vi "Error Handler.vi"(8 "错误输入":cluster{"状态":bool, "代码":i32, "源":string}, 11 "队列输入":refnum<queue>) -> (0 "错误输出":cluster{"状态":bool, "代码":i32, "源":string}, 3 "队列输出":refnum<queue>)   [LabVIEW 2012]
doc: "该子VI监控“生产者循环”和“消费者循环”的“错误簇”连线。任意循环中出错时，该子VI向“消费者循环”发送消息以便关闭循环。"
uses:
  Consumer Message.ctl
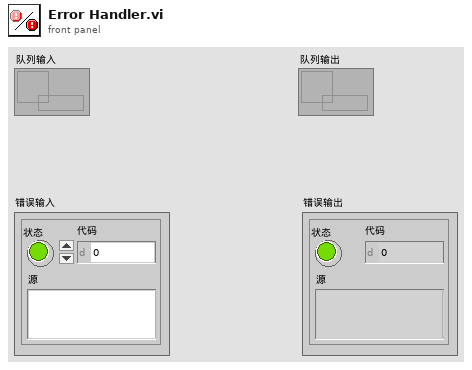
[diagram p1: front panel]
types:
  T1 = typedef "Consumer Message.ctl" = cluster{"消费者状态":string, "布尔数据":bool, "数值数据":i32, "信号":dbl[], "错误":cluster{"状态":bool, "代码":i32, "源":string}}
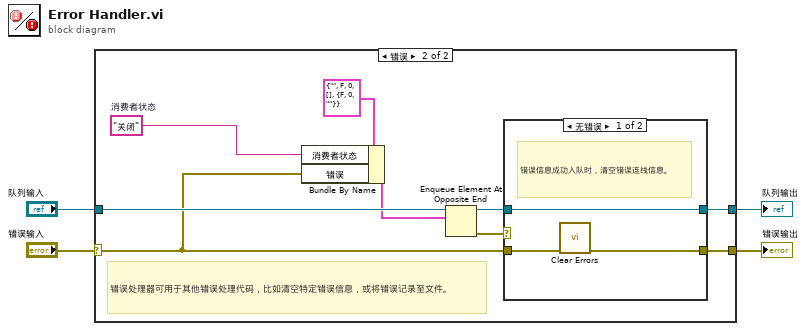
[diagram p0: block diagram]
diagram:
  n1 = case shown="错误" "错误输入" {
    selector: "错误输入" -> [w6 w10]
    tunnel: [w6 w13] -> w3
    tunnel: "队列输入" -> [w5 w15]
    tunnel: [w5 w7] -> w1
    frame No Error {
    }
    frame Error {
      w11 = "关闭"  # 消费者状态
      # "错误处理器可用于其他错误处理代码，比如清空特定错误信息，或将错误记录至文件。"
      n2 = Bundle By Name ("按名称捆绑")(cluster=T1 {"消费者状态"="", "布尔数据"=FALSE, "数值数据"=0, "信号"=[], "错误"={"状态"=FALSE, "代码"=0, "源"=""}}, "消费者状态"=w11, "错误"=w10) -> (w14:T1)
      n3 = Enqueue Element At Opposite End ("队列最前端插入元素")(queue=w15, element=w14) -> (queue out=w8:refnum<queue>, error out=w9:errorcluster)  [unwired: 2 in, 1 out]
      n4 = case shown="无错误" w9 {
        selector: w9 -> [_ w20]
        tunnel: [w18 w20] -> w13
        tunnel: w10 -> [w17 _]
        tunnel: w8 -> [w16 w19]
        tunnel: [w16 w19] -> w7
        frame No Error {
          # "错误信息成功入队时，清空错误连线信息。"
          n5 = call <vilib>:"Clear Errors.vi"("error in (no error)"=w17) -> ("error out"=w18:errorcluster)  [unwired: 6 in]
        }
        frame Error {
          # "如“队列”函数执行失败，则传出错误。"
        }
      }
    }
  }
  "错误输出" <- w3
  "队列输出" <- w1
